vi "RenderJoystickDiagram.vi"(9 "Joystick Graphic Filename":string) -> (1 "Image Out":T1)   [LabVIEW 2023]
doc: "This VI renders a joystick help diagram for display on the dashboard."
uses:
  <vilib>/vision/Image Controls.llb/IMAQ Image.ctl
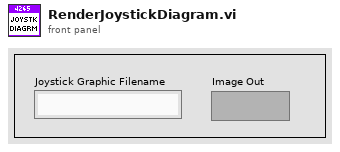
[diagram p1: front panel]
types:
  T1 = typedef "IMAQ Image.ctl" = refnum<image>
  T2 = typedef "imagedata.ctl" = cluster{"image type":i32, "image depth":i32, "image":u8[], "mask":u8[], "colors":u32[], "Rectangle":cluster{"left":i16, "top":i16, "right":i16, "bottom":i16}}
  T3 = typedef "Image Type" = u32
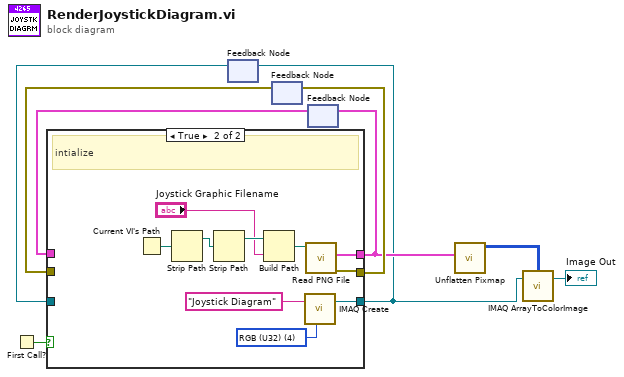
[diagram p0: block diagram]
diagram:
  n1 = First Call?() -> (First Call?: T/F=w9:bool)
  n2 = feedback #1() -> (w8:T1)  [unwired: 1 in]
  n3 = feedback #2() -> (w6:errorcluster)  [unwired: 1 in]
  n4 = feedback #3() -> (w5:T2)  [unwired: 1 in]
  n5 = case shown="True" w9 {
    tunnel: [w12 w20] -> w2
    tunnel: w8 -> [w12 _]
    tunnel: [w11 w14] -> w7
    tunnel: [w10 w13] -> w4
    tunnel: w6 -> [w11 _]
    tunnel: w5 -> [w10 _]
    frame False {
    }
    frame True {
      w21 = T3 4 items=["Grayscale (U8)", "Grayscale (I16)", "Grayscale (SGL)", "Complex (CSG)", "RGB (U32)", "HSL (U32)", "RGB (U64)", "Grayscale (U16)"] ("Image Type")
      # "intialize"
      n6 = Current VI's Path() -> (path=w16:path)
      n7 = Strip Path(path=w16) -> (stripped path=w17:path)  [unwired: 1 out]
      n8 = Strip Path(path=w17) -> (stripped path=w19:path)  [unwired: 1 out]
      n9 = Build Path(base path=w19, name or relative path="Joystick Graphic Filename") -> (appended path=w18:path)
      n10 = call "IMAQ Create"("Image Name"="Joystick Diagram", "Image Type"=w21) -> ("New Image"=w20:T1)  [unwired: 3 in, 1 out]
      n11 = call <vilib>:"Read PNG File.vi"("path to PNG file"=w18) -> ("error out"=w14:errorcluster, "image data"=w13:T2)  [unwired: 8 in, 1 out]
    }
  }
  n12 = feedback-in #1(w2) -> ()
  n13 = feedback-in #2(w7) -> ()
  n14 = feedback-in #3(w4) -> ()
  n15 = call <vilib>:"Unflatten Pixmap.vi"("image data"=w4) -> ("24-bit pixmap"=w3:u32[][])  [unwired: 4 in, 6 out]
  n16 = call "IMAQ ArrayToColorImage"("Image Pixels (U32)"=w3, "Image"=w2) -> ("Image Out"=→"Image Out":T1)  [unwired: 3 in, 1 out]
